vi "XY Graph Get Plots to Preserve.vi"(8 "Error In":errorcluster, 10 "Default (none)":i32[](array[numeric]), 11 "XYGraph in":T1) -> (0 "Error Out":errorcluster, 1 "Preserved Plots Found?":bool, 2 "Preserved Plots":i32[](array[numeric]), 3 "XYGraph out":T1)   [LabVIEW 2019, in "XY Graph Add-Ons.lvlib"]
uses:
  XY Graph Add-Ons.lvlib
  XY Graph Refnum.ctl
  XY Graph Property Tag List.ctl
  <vilib>/UserTags/UserTags.lvlib
  Variant to Data.lvlib
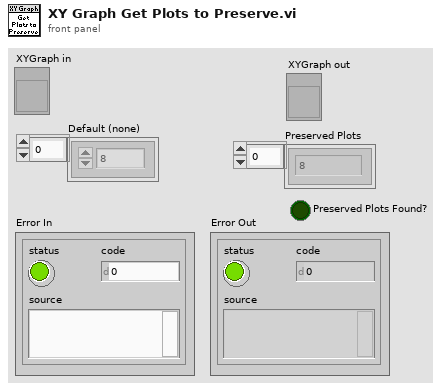
[diagram p1: front panel]
types:
  T1 = typedef "XY Graph Add-Ons.lvlib/XY Graph Refnum.ctl" = refnum<vi>
  T2 = typedef "XY Graph Add-Ons.lvlib/XY Graph Property Tag List.ctl" = enum16{"Max Legend Size", "Preserved Plots", "XScales.GridColors", "YScales.GridColors", "TipStrip String", "TipStrip Visible", "Tool Panels Visibility", "Plots Metadata"}
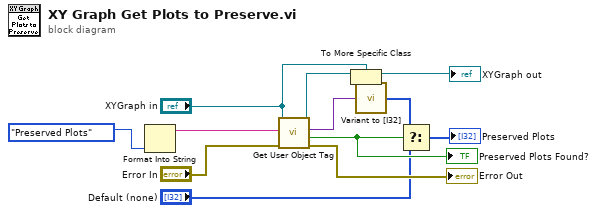
[diagram p0: block diagram]
diagram:
  n1 = Format Into String(XY_Graph_Property_Tag_List."Preserved Plots" ("XY Graph Property Tag")) -> (resulting string=w1:string)  [unwired: 3 in, 1 out]
  n2 = call <vilib>:"Get User Object Tag.vi"("error in (no error)"="Error In", "Tag Name"=w1, "Generic Refnum"="XYGraph in") -> ("error out"=→"Error Out":errorcluster, "Was Tag Found?"=w7:bool, "Value"=w10:variant, "dup Generic Refnum"=w5:refnum<vi>)  [unwired: 5 in]
  "Preserved Plots Found?" <- w7
  n3 = To More Specific Class(target class="XYGraph in", reference=w5) -> (specific class reference=→"XYGraph out":T1)  [unwired: 1 in, 1 out]
  n4 = call "Variant to [I32].vi"("Variant"=w10) -> ("Value"=w9:i32[])  [unwired: 8 in]
  n5 = Select(t=w9, s=w7, f="Default (none)") -> (s? t:f=→"Preserved Plots":i32[])
